vi "303_Module-DeviceSettings_Load.vi"() -> ()   [LabVIEW 2009]
uses:
  <instrlib>/Zurich Instruments LabOne/Public/Modules/ziTypeModEnum.ctl
  <instrlib>/Zurich Instruments LabOne/Public/Modules/ziModSetValueBinary.vi
  <instrlib>/Zurich Instruments LabOne/Zurich Instruments LabOne.lvlib
panel:
  in  "filename":string="MySettingsFile"
  in  "Path":string="C:\\MyFolder"
  out "Connected?":bool=TRUE
  out "Error Out":errorcluster
  in  "Address":string="DEV"
  # "LabOne Modules \nDeviceSettings - Load\nThis VI shows how to load the instrument settings with the xml file. The file can be generated with the L1 user interface in a browser or with any other API using the settings module.\n\nSee block diagram for the VI description.\n\nRequirements: Any Zurich Instrument Product\n\nTo run:\n1. Save a settings file using the LabOne user interface\n2.  Type the path of the folder the setting file is saved.\n3. Type the file name. Do not include .xml file name extension. \n\nTested Devices:\n- HF2LI\n- UHFLI\n- MFLI\n\n\n(c) Zurich Instruments.  ALL RIGHTS RESERVED."
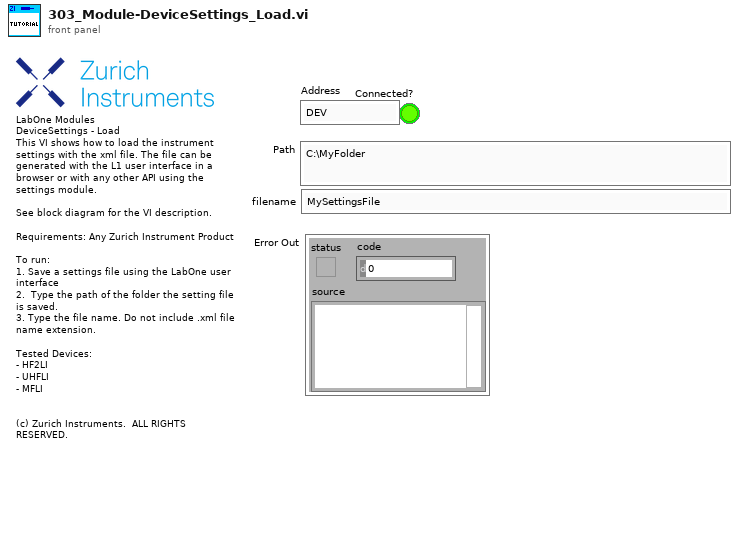
[diagram p1: front panel]
types:
  T1 = typedef "Zurich Instruments LabOne.lvlib/ziTypeModEnum.ctl" = u16
  T2 = typedef "Zurich Instruments LabOne.lvlib/ziTypeHandle.ctl" = cluster{"handleValid":bool, "Conn":u64, "Path Prefix":string, "Handle":u64, "Connected":bool, "Clockbase(s)":dbl}
  T3 = typedef "Zurich Instruments LabOne.lvlib/ziTypeModHandle.ctl" = cluster{"handleValid":bool, "Conn":u64, "ModHandle":u64, "moduleID":string, "Path Prefix":string}
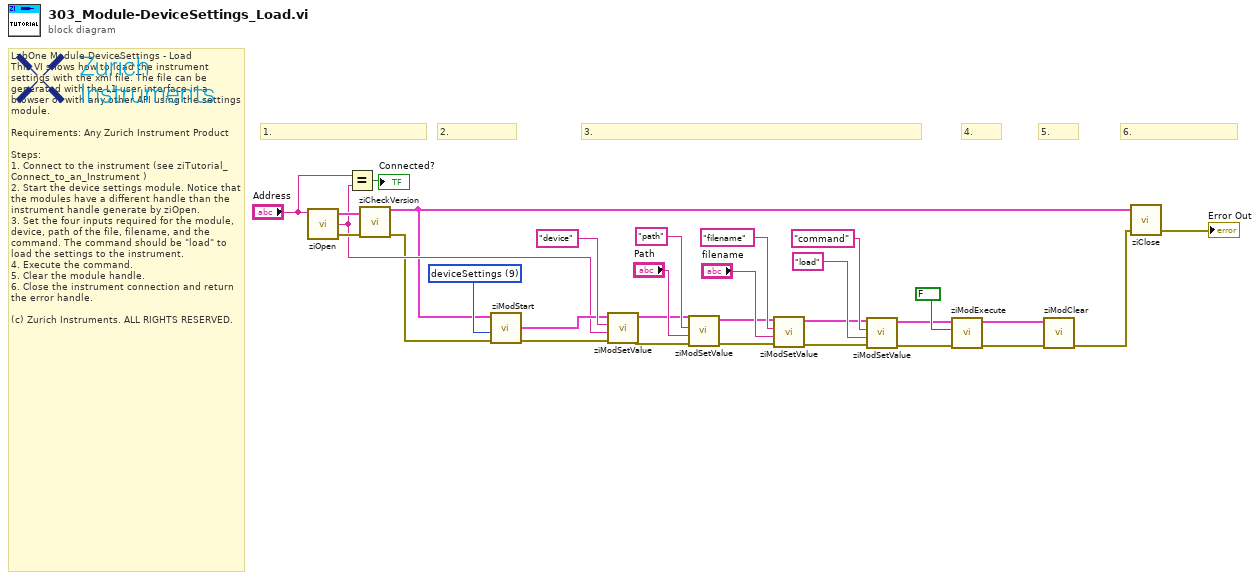
[diagram p0: block diagram]
diagram:
  w16 = T1 9 items=["sweep", "scopeModule", "dataAcquisitionModule", "pidAdvisor", "awgModule", "impedanceModule", "multiDeviceSyncModule", "zoomFFT", "trigger", "deviceSettings", "record", "precompensationAdvisor"] ("module Id")
  # "4."
  # "5."
  # "3."
  # "2."
  # "1."
  # "6."
  # "LabOne Module DeviceSettings - Load\nThis VI shows how to load the instrument settings with the xml file. The file can be generated with the L1 user interface in a browser or with any other API using the settings module.\n\nRequirements: Any Zurich Instrument Product\n\nSteps:\n1. Connect to the instrument (see ziTutorial_Connect_to_an_Instrument )\n2. Start the device settings module. Notice that the modules have a different handle than the instrument handle generate by ziOpen. \n3. Set the four inputs required for the module, device, path of the file, filename, and the command. The command should be \"load\" to load the settings to the instrument.\n4. Execute the command.\n5. Clear the module handle. \n6. Close the instrument connection and return the error handle.\n\n(c) Zurich Instruments. ALL RIGHTS RESERVED."
  n1 = call <instrlib>:"ziOpen.vi"("Address"="Address") -> ("Error Out"=w27:errorcluster, "Selected Device"=w5:string, "HandleOut"=w28:T2)  [unwired: 1 in, 2 out]
  n2 = Equal?(x="Address", y=w5) -> (x = y?=→"Connected?":bool)
  n3 = call <instrlib>:"ziCheckVersion.vi"("Handle In"=w28, "Error In"=w27) -> ("Handle Out"=w1:T2, "Error Out"=w3:errorcluster)  [unwired: 11 in, 1 out]
  n4 = call <instrlib>:"ziModStart.vi"("Error In"=w3, "module Id"=w16, "Handle In"=w1) -> ("Error Out"=w6:errorcluster, "ModHandle Out"=w25:T3)  [unwired: 6 in, 1 out]
  n5 = call-poly <instrlib>:"ziModSetValue.vi"("Error In"=w6, "Data"=w5, "Path"="device", "ModHandle In"=w25) -> ("Error Out"=w13:errorcluster, "ModHandle Out"=w14:T3)  [unwired: 6 in]
  n6 = call-poly <instrlib>:"ziModSetValue.vi"("Error In"=w13, "Data"="Path", "Path"="path", "ModHandle In"=w14) -> ("Error Out"=w17:errorcluster, "ModHandle Out"=w18:T3)  [unwired: 6 in]
  n7 = call-poly <instrlib>:"ziModSetValue.vi"("Error In"=w17, "Data"="filename", "Path"="filename", "ModHandle In"=w18) -> ("Error Out"=w11:errorcluster, "ModHandle Out"=w12:T3)  [unwired: 6 in]
  n8 = call-poly <instrlib>:"ziModSetValue.vi"("Error In"=w11, "Data"="load", "Path"="command", "ModHandle In"=w12) -> ("Error Out"=w9:errorcluster, "ModHandle Out"=w10:T3)  [unwired: 6 in]
  n9 = call <instrlib>:"ziModExecute.vi"("Error In"=w9, "Modal (F)"=FALSE, "ziModHandle In"=w10) -> ("Error Out"=w7:errorcluster, "ziModHandle Out"=w8:T3)  [unwired: 6 in]
  n10 = call <instrlib>:"ziModClear.vi"("Error In"=w7, "ziModHandle In"=w8) -> ("Error Out"=w2:errorcluster)  [unwired: 7 in, 1 out]
  n11 = call <instrlib>:"ziClose.vi"("Error In"=w2, "Handle In"=w1) -> ("Error Out"=→"Error Out":errorcluster)  [unwired: 2 in, 1 out]
